vi "find accumet.vi"() -> (0 "found Accumet":bool, 3 "Serial Port":enum16{"Modem port ", "Printer port"}(ring)=enum."Printer port")   [LabVIEW 2010]
panel:
  in  "ok":bool
  out "message":string="Searching for Accumet..."
  in  "cancel":bool
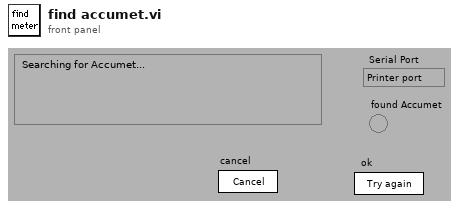
[diagram p1: front panel]
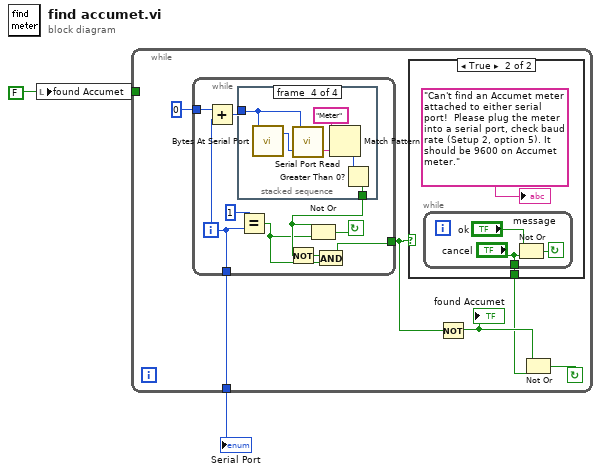
[diagram p0: block diagram]
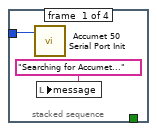
[diagram p2: hidden frame]
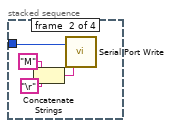
[diagram p3: hidden frame]
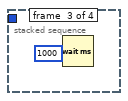
[diagram p4: hidden frame]
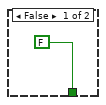
[diagram p5: hidden frame]
diagram:
  w1 = FALSE
  n1 = local write "found Accumet"(w1) -> ()
  n2 = while {
    tunnel: w1 -> [_]
    tunnel: [w7] -> w2
    stop <- w4 continue-if-true
    n3 = while {
      tunnel: [w10] -> w6
      tunnel: 0 -> [w16]
      tunnel: [w15] -> w7
      i -> [w15]
      stop <- w9 continue-if-true
      n4 = Add(x=w16, y=w15) -> (x+y=w14:i32)
      n5 = stacked-sequence {
        tunnel: w14 -> [w19 w23 _ w29]
        tunnel: [_ _ _ w26] -> w13
        frame #0 {
          n6 = call "Accumet 50 Serial Port Init.vi"("port number"=w19) -> ()  [unwired: 6 in, 1 out]
          n7 = local write "message"("Searching for Accumet...") -> ()
        }
        frame #1 {
          n8 = Concatenate Strings("M", "\r") -> (w20:string)
          n9 = call <vilib>:"Serial Port Write.vi"("string to write"=w20, "port number"=w23) -> ()  [unwired: 1 out]
        }
        frame #2 {
          n10 = Wait (ms)(milliseconds to wait=1000) -> ()  [unwired: 1 out]
        }
        frame #3 {
          n11 = call <vilib>:"Bytes At Serial Port.vi"("port number"=w29) -> ("byte count"=w30:u32)  [unwired: 1 out]
          n12 = call <vilib>:"Serial Port Read.vi"("requested byte count"=w30, "port number"=w29) -> ("string read"=w25:string)  [unwired: 1 out]
          n13 = Match Pattern(string=w25, regular expression="Meter") -> (offset past match=w27:i32)  [unwired: 1 in, 3 out]
          n14 = Greater Than 0?(x=w27) -> (x > 0?=w26:bool)
        }
      }
      n15 = Equal?(x=1, y=w15) -> (x = y?=w11:bool)
      n16 = Not(x=w13) -> (.not. x?=w12:bool)
      n17 = Not Or(1:w11, 2:w13) -> (0:w9:bool)
      n18 = And(x=w12, y=w11) -> (x .and. y?=w10:bool)
    }
    n19 = case shown="True" w6 {
      tunnel: [FALSE w32] -> w3
      frame False {
      }
      frame True {
        n20 = while {
          tunnel: ["cancel"] -> w32
          stop <- w35 continue-if-true
          n21 = Not Or(1:"cancel", 2:"ok") -> (0:w35:bool)
        }
        "message" <- "Can't find an Accumet meter attached to either serial port!  Please plug the meter into a serial port, check baud rate (Setup 2, option 5). It should be 9600 on Accumet meter."
      }
    }
    n22 = Not(x=w6) -> (.not. x?=w5:bool)
    "found Accumet" <- w5
    n23 = Not Or(1:w3, 2:w5) -> (0:w4:bool)
  }
  "Serial Port" <- w2
